vi "jsonToStreamCluster.vi"(8 "error in":errorcluster, 11 "jsonConfig":string) -> (0 "error out":errorcluster, 3 "StreamCluster":T1={"DAQ"={"ManagmentRate_Hz"=1, "StreamRate_Hz"=50, "StreamRate_ms"=20, "ManagmentRate_ms"=1000, "refDesArray"=[]}, "Modules"=[]})   [LabVIEW 2024]
uses:
  Control/StreamCluster_TypeDef.ctl
  5f13fa4f-59eb-4706-b0d7-1e32a7d135ec.vi
  78ea79e9-ebde-4a27-bdbc-04c9010114f1.vi
  0b51d5de-1529-409c-bf7e-e6807cdabca0.vi
  5631c9ed-ec5f-4327-9448-355c683cd038.vi
  9ee17ed6-27e4-43bb-8378-30c254ddb443.vi
  b16a306f-ea0e-49ba-9021-b8b6c1909ec0.vi
  b7be143b-341f-4cb6-8338-3b69abefd3c9.vi
  75e0fa59-1fb2-4b06-a272-ca39ac3a5966.vi
  7af6c877-884e-4c12-8d47-110ecfe1d4f4.vi
  d0a09cdd-57ae-44fb-8352-a5f011beae5f.vi
  882ec6e7-461e-45d4-90f9-b5fb31e7bcb1.vi
  e8d8d690-a231-44f6-891b-9ba37c4b53d2.vi
  af8d9ae1-91df-4e32-b776-f5c3ef855bd8.vi
  792fb15a-82a5-4363-8078-894f21c40783.vi
  718e57db-b505-4645-8470-097180e50c55.vi
  ffad590b-2c25-4d0a-9108-e9727b1bec75.vi
  f454ac44-9fbe-4c5b-9868-4bbd337b0ad2.vi
  58d30ee1-9d08-4da1-8002-07e5dbe332a9.vi
  6bdcc115-d705-4e08-be3e-de9065928a61.vi
  751a2d2d-12db-4110-8a63-d3d67d0a3f83.vi
  cdf5def7-eeca-4aee-a50f-e584705918d6.vi
  1eeb4a20-b05c-45b5-9d3d-d1a2408b62a5.vi
  6f47d9fb-de7f-4a71-b63b-0fea03761391.vi
  cd3e4c7d-0f5e-4918-9040-cff85609a479.vi
  <vilib>/JDP Science/JSONtext/Next JSON Value.vi
  <vilib>/JDP Science/JSONtext/String Subset.vi
  <vilib>/JDP Science/JSONtext/Parsing/Advance past next JSON Value (inlined COPY).vi
  <vilib>/JDP Science/JSONtext/Parsing/Advance past whitespace.vi
  <vilib>/JDP Science/JSONtext/Parsing/Advance past String.vi
  <vilib>/JDP Science/JSONtext/Parsing/Advance past Number.vi
  <vilib>/JDP Science/JSONtext/Parsing/Advance past Line Ending.vi
  <vilib>/JDP Science/JSONtext/Parsing/Parse Full Path or Item Name.vi
  <vilib>/JDP Science/JSONtext/Parsing/Advance past Array.vi
  <vilib>/JDP Science/JSONtext/Parsing/Advance past Object.vi
  <vilib>/JDP Science/JSONtext/support/Error Cluster From Code.vi
  <vilib>/JDP Science/JSONtext/Offset/Find Item Locations by Path.vi
  <vilib>/JDP Science/JSONtext/JSON text to Variant.vi
  <vilib>/JDP Science/JSONtext/LVClass Serializer/JSONtext LVClass Serializer.lvclass
  <vilib>/JDP Science/JSONtext/JSONtext.lvlib
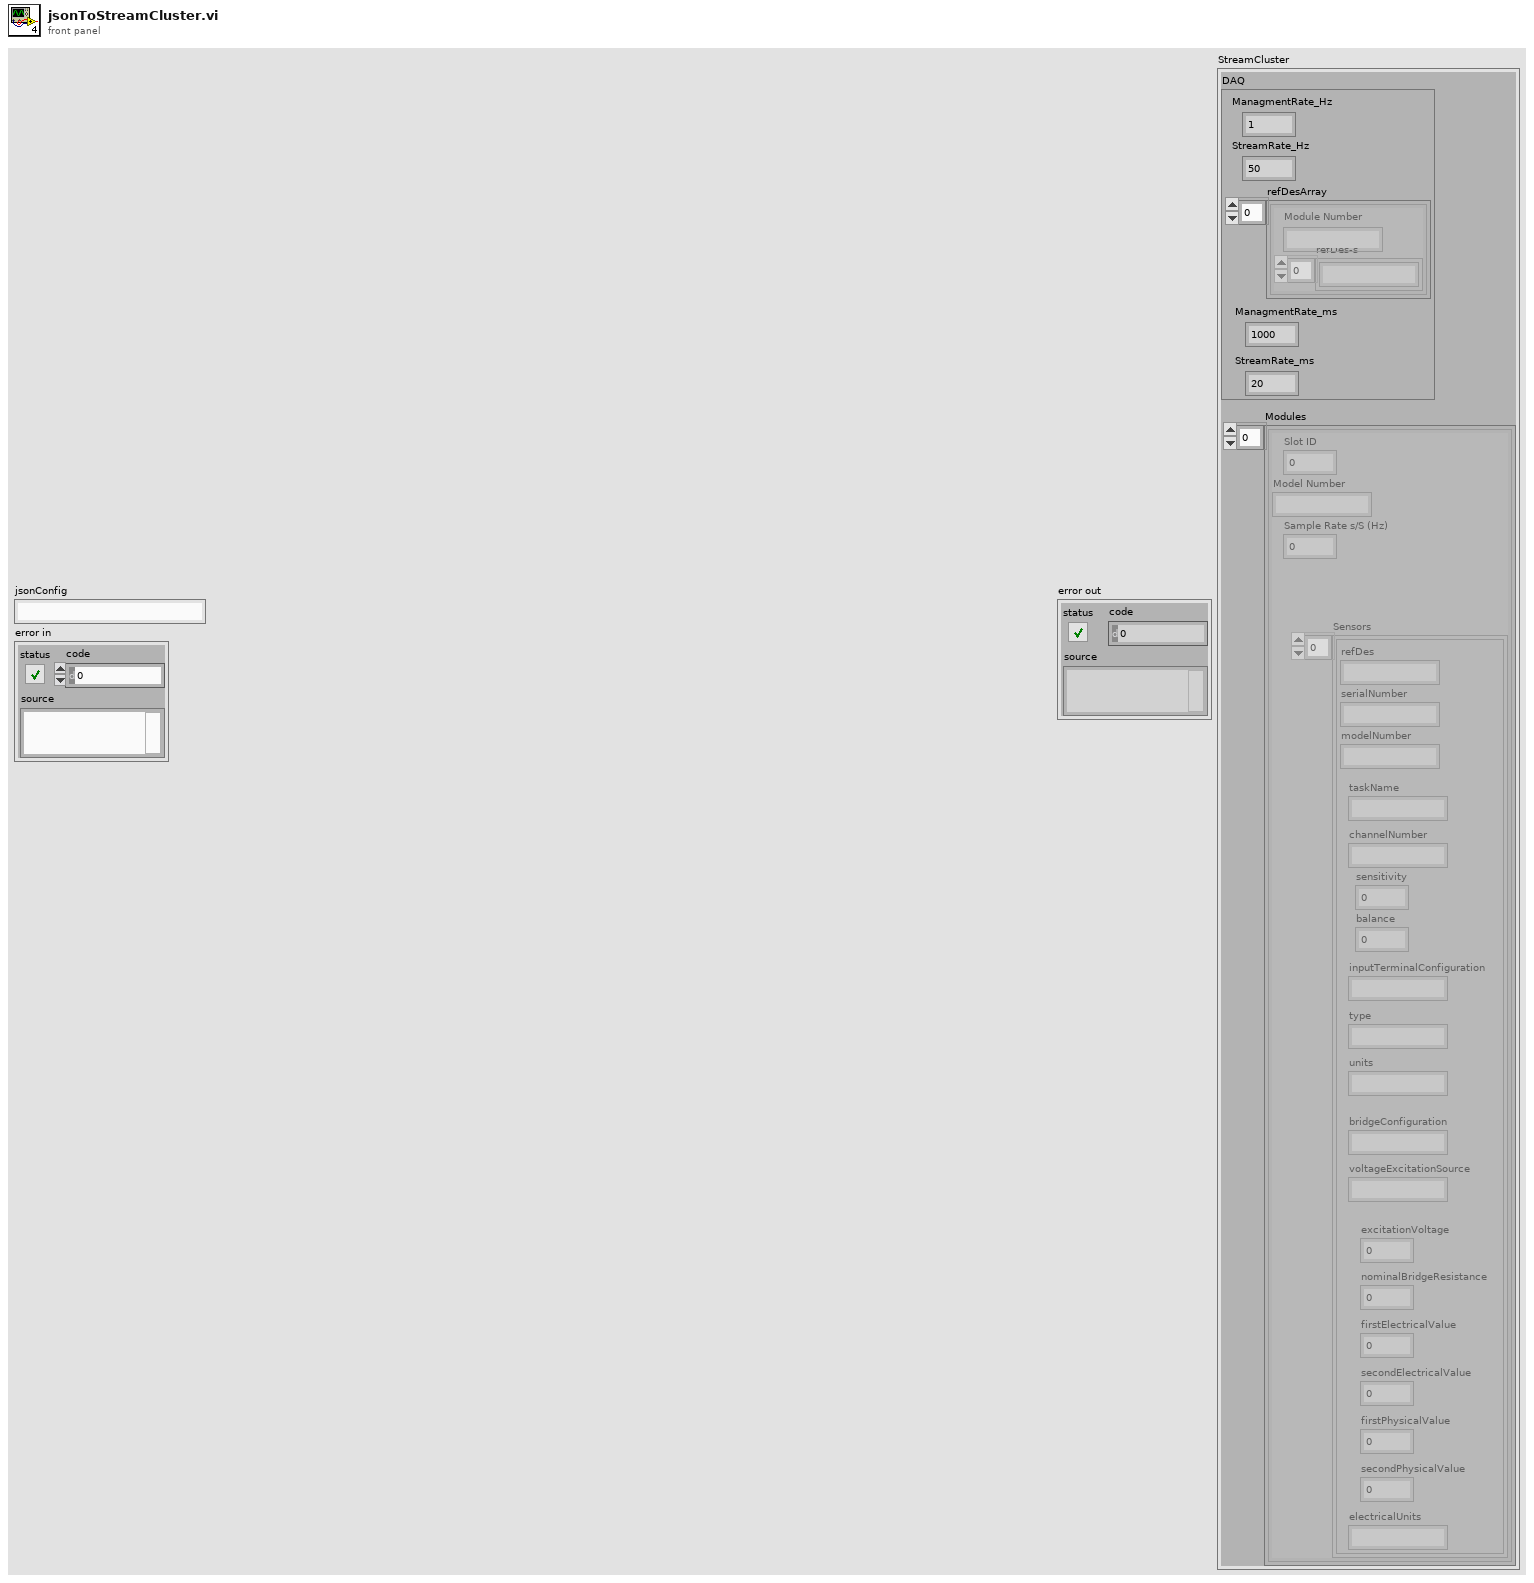
[diagram p1: front panel]
types:
  T1 = typedef "StreamCluster_TypeDef.ctl" = cluster{"DAQ":cluster{"ManagmentRate_Hz":i32, "StreamRate_Hz":i32, "StreamRate_ms":i32, "ManagmentRate_ms":i32, "refDesArray":cluster{"refDes-s":string[], "Module Number":string}[]}, "Modules":cluster{"Slot ID":i32, "Model Number":string, "Sample Rate s/S (Hz)":dbl, "Sensors":cluster{"refDes":string, "serialNumber":string, "modelNumber":string, "units":string, "balance":dbl, "sensitivity":dbl, "type":string, "inputTerminalConfiguration":string, "channelNumber":string, "taskName":string, "bridgeConfiguration":string, "excitationVoltage":dbl, "voltageExcitationSource":string, "nominalBridgeResistance":dbl, "firstElectricalValue":dbl, "secondElectricalValue":dbl, "firstPhysicalValue":dbl, "secondPhysicalValue":dbl, "electricalUnits":string}[]}[]}
  T2 = cluster{"Slot ID":i32, "Model Number":string, "Sample Rate s/S (Hz)":dbl, "Sensors":cluster{"refDes":string, "serialNumber":string, "modelNumber":string, "units":string, "balance":dbl, "sensitivity":dbl, "type":string, "inputTerminalConfiguration":string, "channelNumber":string, "taskName":string, "bridgeConfiguration":string, "excitationVoltage":dbl, "voltageExcitationSource":string, "nominalBridgeResistance":dbl, "firstElectricalValue":dbl, "secondElectricalValue":dbl, "firstPhysicalValue":dbl, "secondPhysicalValue":dbl, "electricalUnits":string}[]}[]
  T3 = cluster{"Slot ID":i32, "Model Number":string, "Sample Rate s/S (Hz)":dbl, "Sensors":cluster{"refDes":string, "serialNumber":string, "modelNumber":string, "units":string, "balance":dbl, "sensitivity":dbl, "type":string, "inputTerminalConfiguration":string, "channelNumber":string, "taskName":string, "bridgeConfiguration":string, "excitationVoltage":dbl, "voltageExcitationSource":string, "nominalBridgeResistance":dbl, "firstElectricalValue":dbl, "secondElectricalValue":dbl, "firstPhysicalValue":dbl, "secondPhysicalValue":dbl, "electricalUnits":string}[]}
  T4 = cluster{"refDes":string, "serialNumber":string, "modelNumber":string, "units":string, "balance":dbl, "sensitivity":dbl, "type":string, "inputTerminalConfiguration":string, "channelNumber":string, "taskName":string, "bridgeConfiguration":string, "excitationVoltage":dbl, "voltageExcitationSource":string, "nominalBridgeResistance":dbl, "firstElectricalValue":dbl, "secondElectricalValue":dbl, "firstPhysicalValue":dbl, "secondPhysicalValue":dbl, "electricalUnits":string}[]
  T5 = cluster{"[0]":string, "[1]":string, "[2]":string, "[3]":string, "[4]":string, "[5]":string, "[6]":string, "[7]":string, "[8]":string, "[9]":string, "[10]":string, "[11]":string, "[12]":string, "[13]":string, "[14]":string, "[15]":string, "[16]":string, "[17]":string, "[18]":string}
  T6 = cluster{"refDes":string, "serialNumber":string, "modelNumber":string, "units":string, "balance":dbl, "sensitivity":dbl, "type":string, "inputTerminalConfiguration":string, "channelNumber":string, "taskName":string, "bridgeConfiguration":string, "excitationVoltage":dbl, "voltageExcitationSource":string, "nominalBridgeResistance":dbl, "firstElectricalValue":dbl, "secondElectricalValue":dbl, "firstPhysicalValue":dbl, "secondPhysicalValue":dbl, "electricalUnits":string}
  T7 = cluster{"[0]":i32, "[1]":i32, "[2]":i32, "[3]":i32, "[4]":i32, "[5]":i32, "[6]":i32, "[7]":i32, "[8]":i32}
  T8 = cluster{"refDes-s":string[], "Module Number":string}[]
  T9 = cluster{"refDes-s":string[], "Module Number":string}
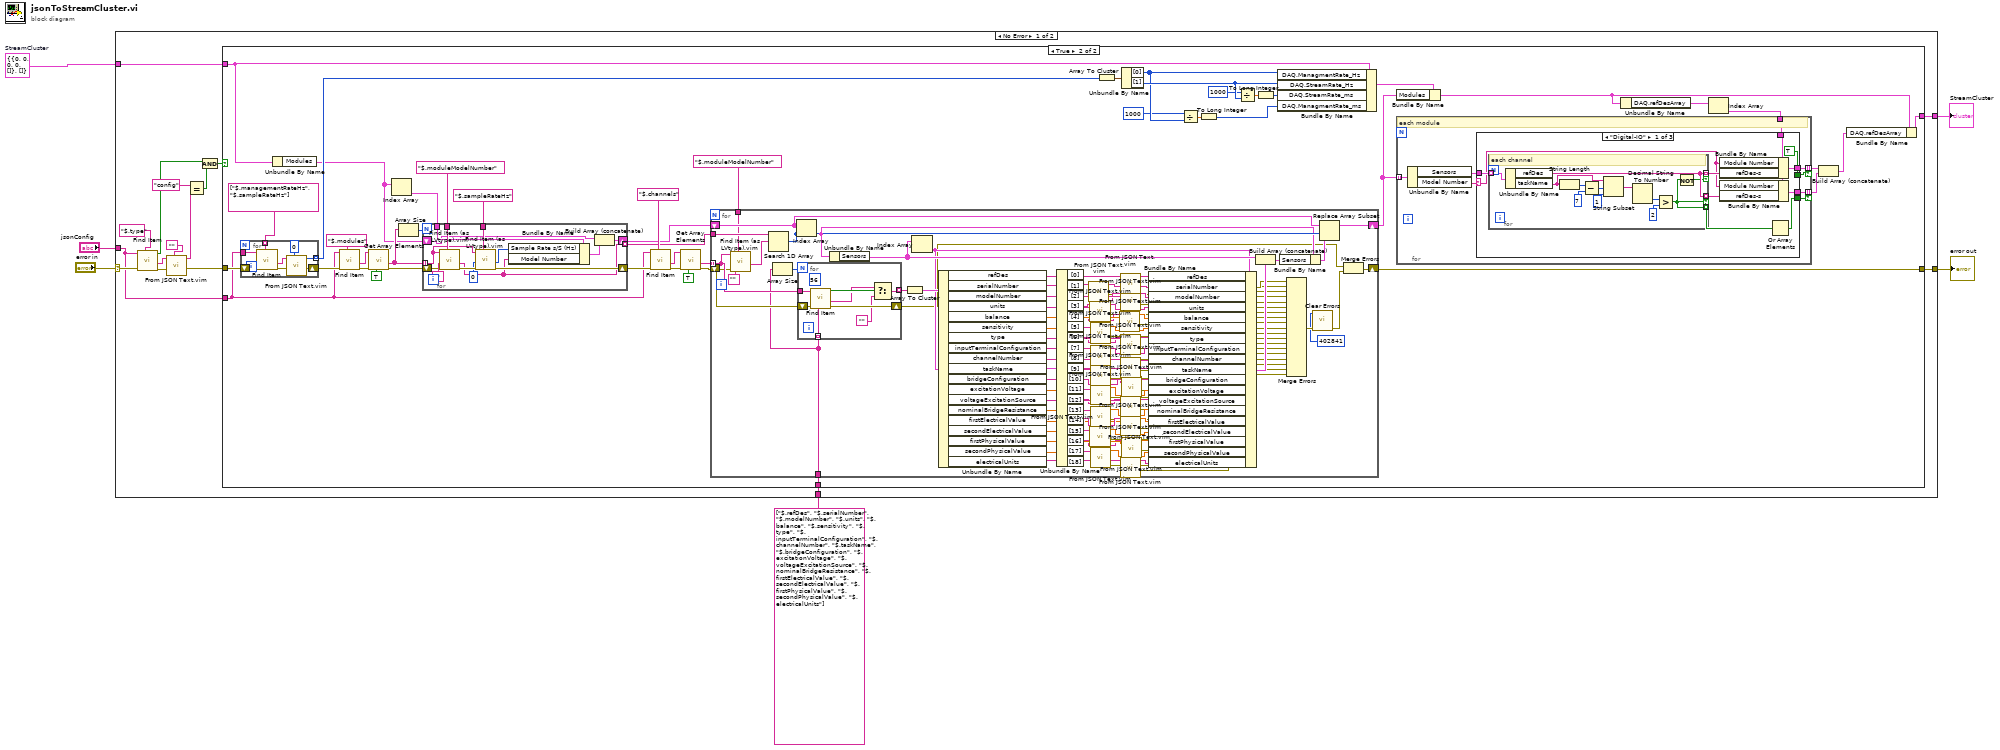
[diagram p0: block diagram]
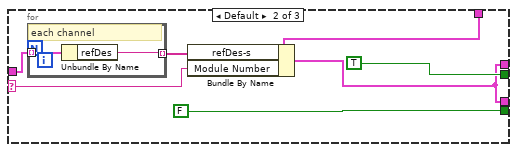
[diagram p3: hidden frame]
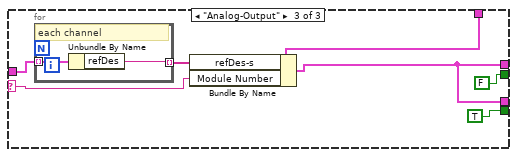
[diagram p4: hidden frame]
diagram:
  w3 = T1 {"DAQ"={"ManagmentRate_Hz"=0, "StreamRate_Hz"=0, "StreamRate_ms"=0, "ManagmentRate_ms"=0, "refDesArray"=[]}, "Modules"=[]}  # StreamCluster
  n1 = case shown="No Error" "error in" {
    selector: "error in" -> [w22 w251]
    tunnel: "jsonConfig" -> [w10 _]
    tunnel: [w8 w251] -> w4
    tunnel: w3 -> [w11 w250]
    tunnel: [w9 w250] -> w1
    tunnel: string[] ["$.refDes", "$.serialNumber", "$.modelNumber", "$.units", "$.balance", "$.sensitivity", "$.type", "$.inputTerminalConfiguration", "$.channelNumber", "$.taskName", "$.bridgeConfiguration", "$.excitationVoltage", "$.voltageExcitationSource", "$.nominalBridgeResistance", "$.firstElectricalValue", "$.secondElectricalValue", "$.firstPhysicalValue", "$.secondPhysicalValue", "$.electricalUnits"] -> [w7 _]
    frame No Error {
      n2 = call <vilib>:"Find Item.vi"("$Path or Item Name"="$.type" ("JSON"), "error in (no error)"=w22, "JSON"=w10) -> ("error out"=w21:errorcluster, "<JSON>"=w20:string, "Found"=w17:bool)  [unwired: 5 in, 1 out]
      n3 = call "From JSON Text.vim"("Data Type and Default Value"="", "error in (no error)"=w21, "JSON"=w20) -> ("error out"=w12:errorcluster, "Data out"=w14:string)  [unwired: 7 in]
      n4 = Equal?(x="config", y=w14) -> (x = y?=w15:bool)
      n5 = Compound Arithmetic op=AND(w17, w15) -> (w16:bool)
      n6 = case shown="True" w16 {
        tunnel: w12 -> [w24 w60]
        tunnel: w11 -> [w23 w59]
        tunnel: w10 -> [_ w45]
        tunnel: [w23 w31] -> w9
        tunnel: [w24 w32] -> w8
        tunnel: w7 -> [_ w34]
        frame False {
        }
        frame True {
          n7 = for {
            shift-right: [w247] -> w57
            shift-left: w60 -> [w249]
            tunnel: [w244] -> w71 mode=indexing
            tunnel: string[] ["$.managementRateHz", "$.sampleRateHz"] -> [w243] mode=indexing
            tunnel: w45 -> [w242]
            n8 = call <vilib>:"Find Item.vi"("$Path or Item Name"=w243, "error in (no error)"=w249, "JSON"=w242) -> ("error out"=w248:errorcluster, "<JSON>"=w245:string)  [unwired: 5 in, 2 out]
            n9 = call "From JSON Text.vim"("Data Type and Default Value"=0, "error in (no error)"=w248, "JSON"=w245) -> ("error out"=w247:errorcluster, "Data out"=w244:i32)  [unwired: 7 in]
          }
          n10 = Unbundle By Name(w59) -> ("Modules"=w38:T2)
          n11 = call <vilib>:"Find Item.vi"("$Path or Item Name"="$.modules", "error in (no error)"=w57, "JSON"=w45) -> ("error out"=w54:errorcluster, "<JSON>"=w53:string)  [unwired: 5 in, 2 out]
          n12 = call <vilib>:"Get Array Elements.vi"("Pass non-arrays"=TRUE, "error in (no error)"=w54, "JSON"=w53) -> ("error out"=w51:errorcluster, "<JSON>"=w39:string[])  [unwired: 6 in, 1 out]
          n13 = Index Array(array=w38) -> (element=w37:T3)  [unwired: 1 in]
          n14 = Array Size(array=w39) -> (size(s)=w40:i32)
          n15 = for {
            N: w40 -> [_]
            tunnel: "$.moduleModelNumber" ("$Path or Item Name") -> [w241]
            tunnel: "$.sampleRateHz" ("$Path or Item Name") -> [w239]
            tunnel: w39 -> [w236] mode=indexing
            shift-right: [w234] -> w46
            shift-left: w51 -> [w235]
            tunnel: [w232] -> w42 mode=indexing
            shift-right: [w228] -> w41
            shift-left: w38 -> [w229]
            tunnel: w37 -> [w231]
            n16 = call "Find Item (as LVtype).vim"("$Path or Item Name"=w241, "error in (no error)"=w235, "Data Type and Default Value"="", "JSON"=w236) -> ("error out"=w238:errorcluster, "Data"=w232:string)  [unwired: 4 in, 2 out]
            n17 = call "Find Item (as LVtype).vim"("$Path or Item Name"=w239, "error in (no error)"=w238, "Data Type and Default Value"=0, "JSON"=w236) -> ("error out"=w234:errorcluster, "Data"=w233:i32)  [unwired: 4 in, 2 out]
            n18 = Bundle By Name(cluster=w231, "Sample Rate s/S (Hz)"=w233, "Model Number"=w232) -> (w230:T3)
            n19 = Build Array (concatenate)(w229, w230) -> (w228:T2)
          }
          n20 = call <vilib>:"Find Item.vi"("$Path or Item Name"="$.channels", "error in (no error)"=w46, "JSON"=w45) -> ("error out"=w49:errorcluster, "<JSON>"=w50:string)  [unwired: 5 in, 2 out]
          n21 = call <vilib>:"Get Array Elements.vi"("Pass non-arrays"=TRUE, "error in (no error)"=w49, "JSON"=w50) -> ("error out"=w44:errorcluster, "<JSON>"=w43:string[])  [unwired: 6 in, 1 out]
          n22 = for {
            shift-right: [w122] -> w32
            shift-left: w44 -> [w208]
            tunnel: w43 -> [w209] mode=indexing
            tunnel: w42 -> [w219]
            shift-right: [w215] -> w33
            shift-left: w41 -> [w216]
            tunnel: "$.moduleModelNumber" -> [w210]
            tunnel: w34 -> [w203]
            n23 = call "Find Item (as LVtype).vim"("$Path or Item Name"=w210, "error in (no error)"=w208, "Data Type and Default Value"="", "JSON"=w209) -> ("Data"=w217:string)  [unwired: 4 in, 3 out]
            n24 = Search 1D Array(1D array=w219, element=w217) -> (index of element=w213:i32)  [unwired: 1 in]
            n25 = Array Size(array=w203) -> (size(s)=w207:i32)
            n26 = Index Array(array=w216, index=w213) -> (element=w212:T3)
            n27 = for {
              N: w207 -> [_]
              tunnel: w209 -> [w227]
              shift-right: [w223] -> w123
              shift-left: w208 -> [w226]
              tunnel: w203 -> [w225] mode=indexing
              tunnel: [w224] -> w206 mode=indexing
              (unwired) 56 ("specific error code to clear (0: all)")
              n28 = call <vilib>:"Find Item.vi"("$Path or Item Name"=w225, "error in (no error)"=w226, "JSON"=w227) -> ("error out"=w223:errorcluster, "<JSON>"=w221:string, "Found"=w222:bool)  [unwired: 5 in, 1 out]
              n29 = Select(t=w221, s=w222, f="") -> (s? t:f=w224:string)
            }
            n30 = Unbundle By Name(w212) -> ("Sensors"=w204:T4)
            n31 = Array To Cluster(array=w206) -> (cluster=w205:T5)
            n32 = Index Array(array=w204) -> (element=w201:T6)  [unwired: 1 in]
            n33 = Unbundle By Name(w201) -> ("refDes"=w199:string, "serialNumber"=w197:string, "modelNumber"=w195:string, "units"=w192:string, "balance"=w188:dbl, "sensitivity"=w185:dbl, "type"=w182:string, "inputTerminalConfiguration"=w179:string, "channelNumber"=w177:string, "taskName"=w174:string, "bridgeConfiguration"=w170:string, "excitationVoltage"=w167:dbl, "voltageExcitationSource"=w165:string, "nominalBridgeResistance"=w161:dbl, "firstElectricalValue"=w158:dbl, "secondElectricalValue"=w155:dbl, "firstPhysicalValue"=w152:dbl, "secondPhysicalValue"=w149:dbl, "electricalUnits"=w146:string)
            n34 = Unbundle By Name(w205) -> ("[0]"=w200:string, "[1]"=w198:string, "[2]"=w194:string, "[3]"=w191:string, "[4]"=w187:string, "[5]"=w186:string, "[6]"=w181:string, "[7]"=w180:string, "[8]"=w176:string, "[9]"=w173:string, "[10]"=w171:string, "[11]"=w168:string, "[12]"=w164:string, "[13]"=w162:string, "[14]"=w159:string, "[15]"=w156:string, "[16]"=w151:string, "[17]"=w150:string, "[18]"=w145:string)
            n35 = call "From JSON Text.vim"("Data Type and Default Value"=w197, "JSON"=w198) -> ("error out"=w143:errorcluster, "Data out"=w196:string)  [unwired: 8 in]
            n36 = call "From JSON Text.vim"("Data Type and Default Value"=w192, "JSON"=w191) -> ("error out"=w141:errorcluster, "Data out"=w190:string)  [unwired: 8 in]
            n37 = call "From JSON Text.vim"("Data Type and Default Value"=w155, "JSON"=w156) -> ("error out"=w129:errorcluster, "Data out"=w154:dbl)  [unwired: 8 in]
            n38 = call "From JSON Text.vim"("Data Type and Default Value"=w185, "JSON"=w186) -> ("error out"=w139:errorcluster, "Data out"=w184:dbl)  [unwired: 8 in]
            n39 = call "From JSON Text.vim"("Data Type and Default Value"=w179, "JSON"=w180) -> ("error out"=w137:errorcluster, "Data out"=w178:string)  [unwired: 8 in]
            n40 = call "From JSON Text.vim"("Data Type and Default Value"=w174, "JSON"=w173) -> ("error out"=w135:errorcluster, "Data out"=w172:string)  [unwired: 8 in]
            n41 = call "From JSON Text.vim"("Data Type and Default Value"=w167, "JSON"=w168) -> ("error out"=w133:errorcluster, "Data out"=w166:dbl)  [unwired: 8 in]
            n42 = call "From JSON Text.vim"("Data Type and Default Value"=w161, "JSON"=w162) -> ("error out"=w131:errorcluster, "Data out"=w160:dbl)  [unwired: 8 in]
            n43 = call "From JSON Text.vim"("Data Type and Default Value"=w149, "JSON"=w150) -> ("error out"=w126:errorcluster, "Data out"=w148:dbl)  [unwired: 8 in]
            n44 = call "From JSON Text.vim"("Data Type and Default Value"=w188, "JSON"=w187) -> ("error out"=w140:errorcluster, "Data out"=w189:dbl)  [unwired: 8 in]
            n45 = call "From JSON Text.vim"("Data Type and Default Value"=w199, "JSON"=w200) -> ("error out"=w144:errorcluster, "Data out"=w120:string)  [unwired: 8 in]
            n46 = call "From JSON Text.vim"("Data Type and Default Value"=w195, "JSON"=w194) -> ("error out"=w142:errorcluster, "Data out"=w193:string)  [unwired: 8 in]
            n47 = call "From JSON Text.vim"("Data Type and Default Value"=w182, "JSON"=w181) -> ("error out"=w138:errorcluster, "Data out"=w183:string)  [unwired: 8 in]
            n48 = call "From JSON Text.vim"("Data Type and Default Value"=w177, "JSON"=w176) -> ("error out"=w136:errorcluster, "Data out"=w175:string)  [unwired: 8 in]
            n49 = call "From JSON Text.vim"("Data Type and Default Value"=w165, "JSON"=w164) -> ("error out"=w132:errorcluster, "Data out"=w163:string)  [unwired: 8 in]
            n50 = call "From JSON Text.vim"("Data Type and Default Value"=w158, "JSON"=w159) -> ("error out"=w130:errorcluster, "Data out"=w157:dbl)  [unwired: 8 in]
            n51 = call "From JSON Text.vim"("Data Type and Default Value"=w146, "JSON"=w145) -> ("error out"=w127:errorcluster, "Data out"=w147:string)  [unwired: 8 in]
            n52 = call "From JSON Text.vim"("Data Type and Default Value"=w170, "JSON"=w171) -> ("error out"=w134:errorcluster, "Data out"=w169:string)  [unwired: 8 in]
            n53 = call "From JSON Text.vim"("Data Type and Default Value"=w152, "JSON"=w151) -> ("error out"=w128:errorcluster, "Data out"=w153:dbl)  [unwired: 8 in]
            n54 = Bundle By Name(cluster=w201, "refDes"=w120, "serialNumber"=w196, "modelNumber"=w193, "units"=w190, "balance"=w189, "sensitivity"=w184, "type"=w183, "inputTerminalConfiguration"=w178, "channelNumber"=w175, "taskName"=w172, "bridgeConfiguration"=w169, "excitationVoltage"=w166, "voltageExcitationSource"=w163, "nominalBridgeResistance"=w160, "firstElectricalValue"=w157, "secondElectricalValue"=w154, "firstPhysicalValue"=w153, "secondPhysicalValue"=w148, "electricalUnits"=w147) -> (w202:T6)
            n55 = Build Array (concatenate)(w204, w202) -> (w211:T4)
            n56 = Bundle By Name(cluster=w212, "Sensors"=w211) -> (w214:T3)
            n57 = Merge Errors(w144, w143, w142, w141, w140, w139, w138, w137, w136, w135, w134, w133, w132, w131, w130, w129, w128, w126, w127) -> (w125:errorcluster)
            n58 = call <vilib>:"Clear Errors.vi"("error in (no error)"=w125, "specific error code to clear (0: all)"=402841) -> ("error out"=w121:errorcluster)  [unwired: 4 in, 1 out]
            n59 = Replace Array Subset(array=w216, new element=w214, index=w213) -> (w215:T2)
            n60 = Merge Errors(w123, w121) -> (w122:errorcluster)
          }
          n61 = Array To Cluster(array=w71) -> (cluster=w64:T7)
          n62 = Unbundle By Name(w64) -> ("[0]"=w67:i32, "[1]"=w70:i32)
          n63 = Divide(x=1000, y=w67) -> (x/y=w65:dbl)
          n64 = To Long Integer(number=w65) -> (32bit integer=w66:i32)
          n65 = Divide(x=1000, y=w70) -> (x/y=w68:dbl)
          n66 = To Long Integer(number=w68) -> (32bit integer=w69:i32)
          n67 = Bundle By Name(cluster=w59, "DAQ.ManagmentRate_Hz"=w67, "DAQ.StreamRate_Hz"=w70, "DAQ.StreamRate_ms"=w69, "DAQ.ManagmentRate_ms"=w66) -> (w35:T1)
          n68 = Bundle By Name(cluster=w35, "Modules"=w33) -> (w27:T1)
          n69 = Unbundle By Name(w27) -> ("DAQ.refDesArray"=w26:T8)
          n70 = Index Array(array=w26) -> (element=w25:T9)  [unwired: 1 in]
          n71 = for {
            tunnel: w33 -> [w73] mode=indexing
            tunnel: [w78] -> w30 mode=indexing if=w74
            tunnel: [w76] -> w29 mode=indexing if=w75
            tunnel: w25 -> [w72]
            # "each module"
            n72 = Unbundle By Name(w73) -> ("Sensors"=w79:T4, "Model Number"=w77:string)
            n73 = case shown="\"Digital-IO\"" w77 {
              selector: w77 -> [w80 w102 w113]
              tunnel: w79 -> [w89 w108 w117]
              tunnel: [w85 w105 w111] -> w78
              tunnel: [w82 w105 w111] -> w76
              tunnel: [w87 FALSE TRUE] -> w75
              tunnel: [TRUE TRUE FALSE] -> w74
              tunnel: w72 -> [w81 w104 w112]
              frame "Digital-IO" {
                n74 = for {
                  tunnel: w89 -> [w101] mode=indexing
                  tunnel: [w100] -> w84 mode=indexing if=w92
                  tunnel: [w100] -> w83 mode=indexing if=w91
                  tunnel: [w91] -> w88 mode=indexing
                  # "each channel"
                  n75 = Unbundle By Name(w101) -> ("refDes"=w100:string, "taskName"=w90:string)
                  n76 = String Length(string=w90) -> (length=w99:i32)
                  n77 = Subtract(x=w99, y=7) -> (x-y=w97:i32)
                  n78 = String Subset(string=w90, offset (0)=w97, length (rest)=1 ("length (rest)")) -> (substring=w95:string)
                  n79 = Decimal String To Number(string=w95) -> (number=w94:i32)  [unwired: 2 in, 1 out]
                  n80 = Greater?(x=w94, y=2) -> (0:w91:bool)
                  n81 = Not(x=w91) -> (.not. x?=w92:bool)
                }
                n82 = Bundle By Name(cluster=w81, "Module Number"=w80, "refDes-s"=w84) -> (w85:T9)
                n83 = Bundle By Name(cluster=w81, "Module Number"=w80, "refDes-s"=w83) -> (w82:T9)
                n84 = Or Array Elements(Boolean array=w88) -> (logical OR=w87:bool)
              }
              frame Default {
                n85 = for {
                  tunnel: w108 -> [w110] mode=indexing
                  tunnel: [w109] -> w103 mode=indexing
                  # "each channel"
                  n86 = Unbundle By Name(w110) -> ("refDes"=w109:string)
                }
                n87 = Bundle By Name(cluster=w104, "refDes-s"=w103, "Module Number"=w102) -> (w105:T9)
              }
              frame "Analog-Output" {
                n88 = for {
                  tunnel: w117 -> [w119] mode=indexing
                  tunnel: [w118] -> w114 mode=indexing
                  # "each channel"
                  n89 = Unbundle By Name(w119) -> ("refDes"=w118:string)
                }
                n90 = Bundle By Name(cluster=w112, "refDes-s"=w114, "Module Number"=w113) -> (w111:T9)
              }
            }
          }
          n91 = Build Array (concatenate)(w30, w29) -> (w28:T8)
          n92 = Bundle By Name(cluster=w27, "DAQ.refDesArray"=w28) -> (w31:T1)
        }
      }
    }
    frame Error {
    }
  }
  "error out" <- w4
  "StreamCluster" <- w1
